vi "formattitel&showannotation.vi"(0 "reference":refnum<vi>) -> ()   [LabVIEW 2012]
uses:
  System.Windows.Forms
  musicplayer_glo.vi
  player_glo.vi
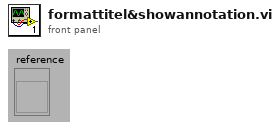
[diagram p1: front panel]
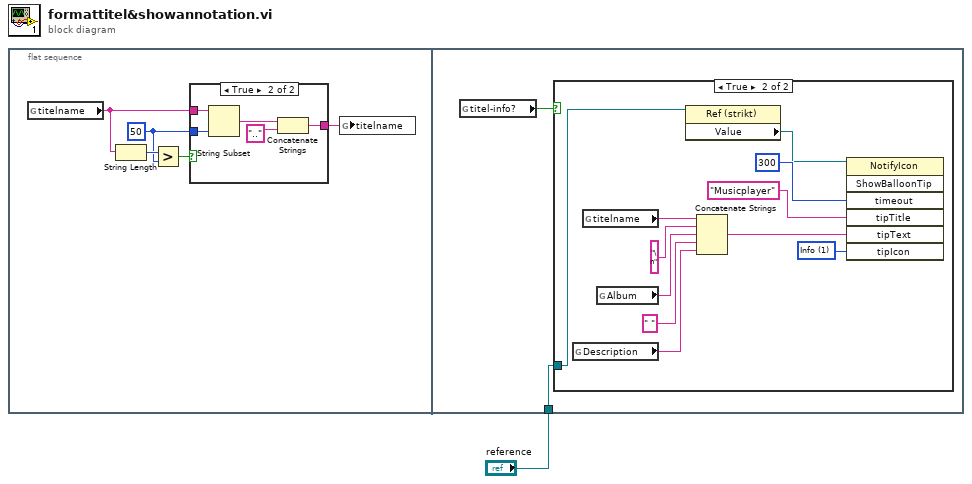
[diagram p0: block diagram]
diagram:
  n1 = flat-sequence {
    tunnel: "reference" -> [w13]
    frame #0 {
      w4 = 50 ("y")
      n2 = global read "musicplayer_glo.vi" "titelname"() -> (w3:string)
      n3 = String Length(string=w3) -> (length=w6:i32)
      n4 = Greater?(x=w6, y=w4) -> (0:w5:bool)
      n5 = case shown="True" w5 {
        tunnel: w3 -> [w7 w11]
        tunnel: [w7 w8] -> w2
        tunnel: w4 -> [_ w12]
        frame False {
        }
        frame True {
          n6 = String Subset(string=w11, length (rest)=w12) -> (substring=w9:string)  [unwired: 1 in]
          n7 = Concatenate Strings(w9, ".." ("String")) -> (w8:string)
        }
      }
      n8 = global write "musicplayer_glo.vi" "titelname"(w2) -> ()
    }
    frame #1 {
      n9 = global read "musicplayer_glo.vi" "titel-info?"() -> (w14:bool)
      n10 = case shown="True" w14 {
        tunnel: w13 -> [_ w15]
        frame False {
        }
        frame True {
          w24 = 1 items=["None", "Info", "Warning", "Error"] ("tipIcon")
          n11 = global read "player_glo.vi" "Description"() -> (w16:string)
          n12 = global read "musicplayer_glo.vi" "titelname"() -> (w20:string)
          n13 = global read "player_glo.vi" "Album"() -> (w18:string)
          n14 = property class="Ref (strikt)"(reference=w15) -> ("Value"=w21:refnum<k24>)  [unwired: 1 in, 2 out]
          n15 = Concatenate Strings(w20, "\n" ("String"), w18, " " ("String"), w16) -> (w25:string)
          n16 = invoke class="NotifyIcon" method="ShowBalloonTip"(reference=w21, "timeout"=300, "tipTitle"="Musicplayer", "tipText"=w25, "tipIcon"=w24) -> ()  [unwired: 2 in, 7 out]
        }
      }
    }
  }
